vi "正常显示转十六进制显示 (子VI).vi"(11 "字符串输入":string) -> (3 "字符串输出":string)   [LabVIEW 2016, in "环境动力监测库.lvlib"]
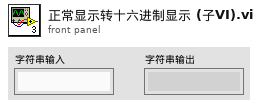
[diagram p1: front panel]
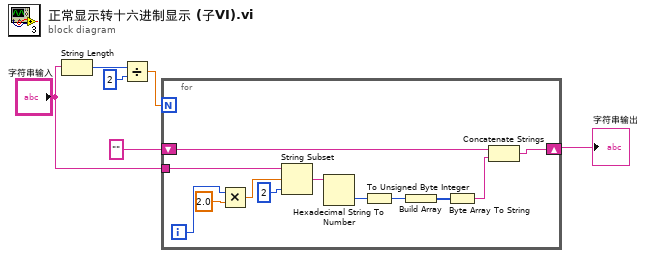
[diagram p0: block diagram]
diagram:
  n1 = String Length(string="字符串输入") -> (length=w1:i32)
  n2 = Divide(x=w1, y=2) -> (x/y=w3:dbl)
  n3 = for {
    N: w3 -> [_]
    shift-right: [w9] -> w5
    shift-left: "" -> [w10]
    tunnel: "字符串输入" -> [w8]
    i -> [w7]
    n4 = Multiply(x=w7, y=2.0) -> (x*y=w13:dbl)
    n5 = String Subset(string=w8, offset (0)=w13, length (rest)=2 ("长度（剩余）")) -> (substring=w12:string)
    n6 = Hexadecimal String To Number(string=w12) -> (number=w17:u32)  [unwired: 2 in, 1 out]
    n7 = To Unsigned Byte Integer(number=w17) -> (unsigned 8bit integer=w16:u8)
    n8 = Build Array(w16) -> (w18:u8[])
    n9 = Byte Array To String(unsigned byte array=w18) -> (string=w11:string)
    n10 = Concatenate Strings(w10, w11) -> (w9:string)
  }
  "字符串输出" <- w5
